vi "AutonDrive Test.vi"() -> ()   [LabVIEW 2014]
panel:
  in  "Feet":dbl=1.0 format="%#_13g"
  in  "Boolean":bool
  out "Distance (ft)":dbl(knob) scale=0.0..10.0
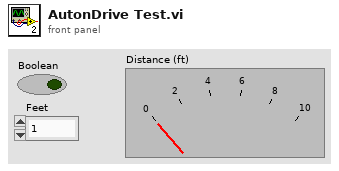
[diagram p1: front panel]
types:
  T1 = enum16{"Move Forward", "Move Backward", "Strafe Right", "Strafe Left"}
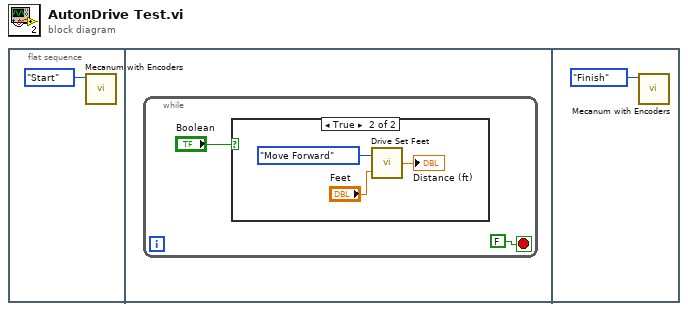
[diagram p0: block diagram]
diagram:
  n1 = flat-sequence {
    frame #0 {
      n2 = call "Mecanum with Encoders.vi"("Mode"=enum8{"Start", "Run", "Finish"}."Start") -> ()  [unwired: 9 in, 1 out]
    }
    frame #1 {
      n3 = while {
        stop <- FALSE stop-if-true
        n4 = case shown="True" "Boolean" {
          frame False {
          }
          frame True {
            n5 = call "Drive Set Feet.vi"("Feet"="Feet", "Direction"=T1."Move Forward") -> ("Distance (ft)"=→"Distance (ft)":dbl)
          }
        }
      }
    }
    frame #2 {
      n6 = call "Mecanum with Encoders.vi"("Mode"=enum8{"Start", "Run", "Finish"}."Finish") -> ()  [unwired: 9 in, 1 out]
    }
  }
